vi "BuildMask.vi"   [LabVIEW 2010]
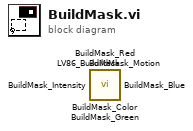
[diagram p0: block diagram]
diagram:
  n1 = call <userlib>:"BuildMask_Color.vi"() -> ()  [unwired: 3 in, 1 out]
  n2 = call <userlib>:"BuildMask_Motion.vi"() -> ()  [unwired: 3 in, 1 out]
  n3 = call <userlib>:"BuildMask_Intensity.vi"() -> ()  [unwired: 3 in, 1 out]
  n4 = call <userlib>:"BuildMask_Blue.vi"() -> ()  [unwired: 3 in, 1 out]
  n5 = call <userlib>:"BuildMask_Green.vi"() -> ()  [unwired: 3 in, 1 out]
  n6 = call <userlib>:"BuildMask_Red.vi"() -> ()  [unwired: 3 in, 1 out]
  n7 = call <userlib>:"LV86_BuildMask.vi"() -> ()  [unwired: 3 in, 1 out]
